vi "parse best fit into string array.vi"(11 "Initial Best Fit":dbl[](array[numeric])=[0.95, 0.7847488427218173, 0.09, 0.95, 0.7805916961729282, 0.04711557674921147, 0.95, 0.8881897967254512, 0.061587383360674375, 0.95, 1.0303480028067902, 0.06277625222382, 0.95, 1.0618615544456425, 0.08999856002359032, 0.95, 1.1217690925, 0.07675393176243342, 0.0, 0.0, 0.0]) -> (3 "concatenated string":string)   [LabVIEW 2016]
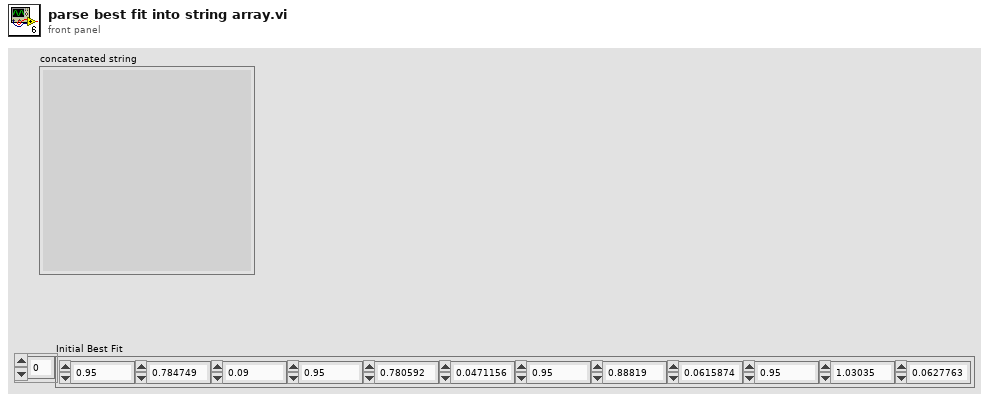
[diagram p1: front panel]
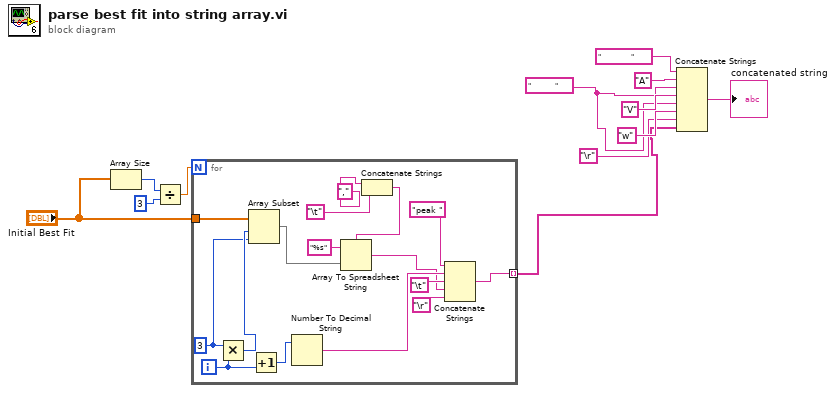
[diagram p0: block diagram]
diagram:
  w1 = "            " ("string")
  n1 = Array Size(array="Initial Best Fit") -> (size(s)=w11:i32)
  n2 = Divide(x=w11, y=3 ("x")) -> (x/y=w9:dbl)
  n3 = for {
    N: w9 -> [_]
    tunnel: "Initial Best Fit" -> [w27]
    tunnel: [w20] -> w3 mode=indexing
    i -> [w22]
    w25 = 3 ("x")
    n4 = Multiply(x=w25, y=w22) -> (x*y=w26:i32)
    n5 = Array Subset(array=w27, index=w26, length=w25) -> (w24:dbl[])
    n6 = Increment(x=w22) -> (x+1=w16:i32)
    n7 = Number To Decimal String(number=w16) -> (decimal integer string=w21:string)  [unwired: 1 in]
    n8 = Concatenate Strings("," ("string"), "\t") -> (w15:string)
    n9 = Array To Spreadsheet String(delimiter (Tab)=w15, array=w24, 3:"%s" ("format string")) -> (spreadsheet string=w18:string)
    n10 = Concatenate Strings("peak ", w21, "\t", w18, "\r") -> (w20:string)
  }
  n11 = Concatenate Strings("               " ("string"), "A" ("string"), w1, "V" ("string"), w1, "w" ("string"), "\r", w3) -> (→"concatenated string":string)
